vi "Open Front Panel.vi"(6 "Custom Window Size":cluster{"Height":i16, "Width":i16}, 8 "error in (no error)":errorcluster, 9 "Custom Window Position":cluster{"Top":i16, "Left":i16}, 10 "Position":T1, 11 "IViewable in":refnum<class "IViewable.lvclass">) -> (0 "error out":errorcluster, 3 "IViewable out":refnum<class "IViewable.lvclass">)   [LabVIEW 2019, in "IViewable.lvlib" / "IViewable.lvclass"]
doc: "<License>\nCopyright © 2017 Composed Systems, LLC | All rights reserved\nwww.composed.io\n\nAuthor: Ethan Stern <ethan.stern@composed.io>\n\nThis software is provided \"AS IS\" WITHOUT WARRANTIES, either express or implied, AND IS FOR EDUCATIONAL PURPOSES ONLY.\n</License>"
uses:
  <vilib>/gpm_packages/@cs/mva-viewable/Source/IViewable/IViewable/IViewable.lvclass
  <vilib>/gpm_packages/@cs/mva-viewable/Source/IViewable/IViewable/View Position Enum.ctl
  <vilib>/gpm_packages/@cs/mva-viewable/Source/IViewable/IViewable/IViewable.lvclass/IViewable.ctl
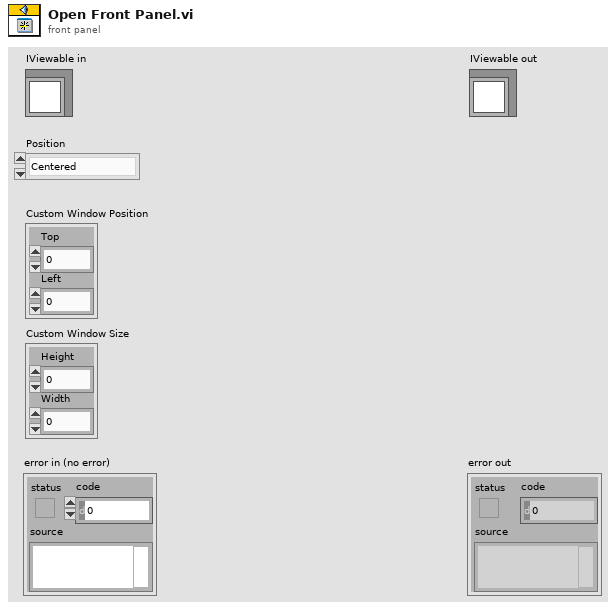
[diagram p1: front panel]
types:
  T1 = typedef "IViewable.lvlib/IViewable.lvclass/View Position Enum.ctl" = enum16{"Centered", "Maximized", "Minimized", "Custom", "Unchanged"}
  T2 = enum32{"Invalid", "Standard", "Closed", "Hidden", "Minimized", "Maximized"}
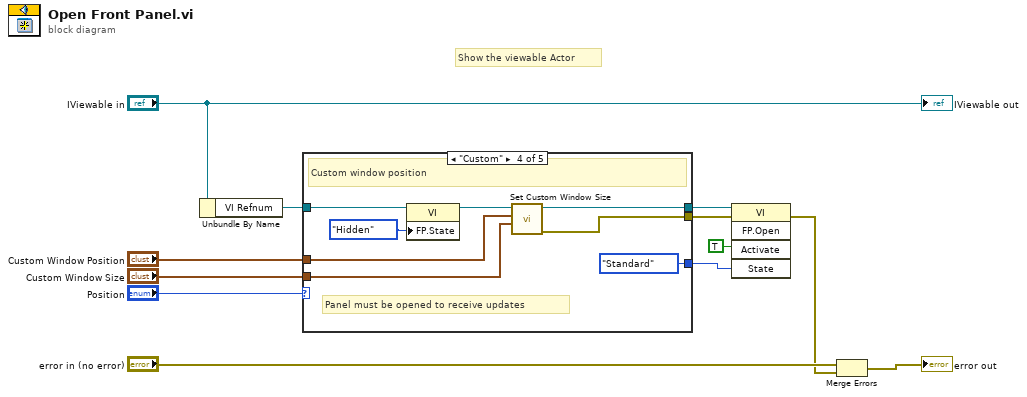
[diagram p0: block diagram]
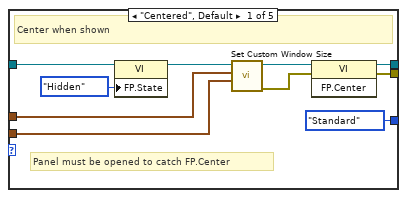
[diagram p2: hidden frame]
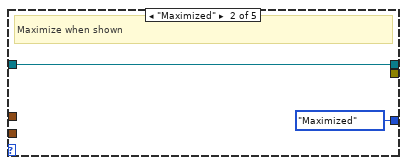
[diagram p3: hidden frame]
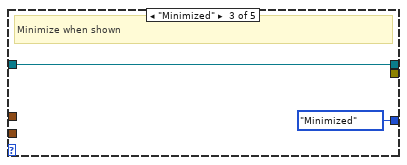
[diagram p4: hidden frame]
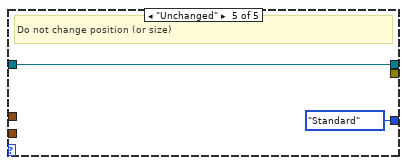
[diagram p5: hidden frame]
diagram:
  # "Show the viewable Actor"
  n1 = Unbundle By Name("IViewable in") -> ("VI Refnum"=w10:refnum<vi>)
  n2 = case shown="\"Custom\"" "Position" {
    tunnel: w10 -> [w22 w24 w26 w29 w36]
    tunnel: [w21 w24 w26 w33 w36] -> w3
    tunnel: [w20 _ _ w32 _] -> w6
    tunnel: "Custom Window Position" -> [w15 _ _ w31 _]
    tunnel: [T2."Standard" ("State") T2."Maximized" ("State") T2."Minimized" ("State") T2."Standard" ("State") T2."Standard" ("State")] -> w4
    tunnel: "Custom Window Size" -> [w14 _ _ w30 _]
    frame "Centered", Default {
      # "Panel must be opened to catch FP.Center"
      # "Center when shown"
      n3 = property class="VI"(reference=w22, "FP.State"=T2."Hidden" ("Front Panel Window:State")) -> (reference out=w18:refnum<vi>)  [unwired: 1 in, 1 out]
      n4 = call <vilib>:"Set Custom Window Size.vi"("Custom Window Size"=w14, "Custom Window Position"=w15, "VI in"=w18) -> ("error out"=w13:errorcluster, "VI out"=w16:refnum<vi>)  [unwired: 7 in]
      n5 = invoke class="VI" method="FP.Center"(reference=w16, error in=w13) -> (reference out=w21:refnum<vi>, error out=w20:errorcluster)  [unwired: 1 in, 1 out]
    }
    frame "Maximized" {
      # "Maximize when shown"
    }
    frame "Minimized" {
      # "Minimize when shown"
    }
    frame "Custom" {
      # "Panel must be opened to receive updates"
      # "Custom window position"
      n6 = property class="VI"(reference=w29, "FP.State"=T2."Hidden" ("Front Panel Window:State")) -> (reference out=w28:refnum<vi>)  [unwired: 1 in, 1 out]
      n7 = call <vilib>:"Set Custom Window Size.vi"("Custom Window Size"=w30, "Custom Window Position"=w31, "VI in"=w28) -> ("error out"=w32:errorcluster, "VI out"=w33:refnum<vi>)  [unwired: 7 in]
    }
    frame "Unchanged" {
      # "Do not change position (or size)"
    }
  }
  n8 = invoke class="VI" method="FP.Open"(reference=w3, error in=w6, "Activate"=TRUE ("Activate?"), "State"=w4) -> (error out=w9:errorcluster)  [unwired: 1 in, 4 out]
  n9 = Merge Errors("error in (no error)", w9) -> (→"error out":errorcluster)
  "IViewable out" <- "IViewable in"
